vi "ModuleMain.vi"(8 "error in (no error)":errorcluster) -> (0 "error out":errorcluster)   [LabVIEW 2017, in "LeapMotion.lvlib"]
doc: "Module Main VI"
uses:
  LeapMotion.lvlib
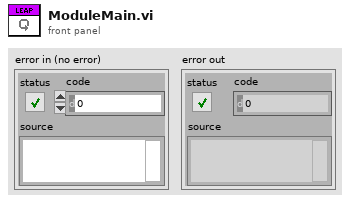
[diagram p1: front panel]
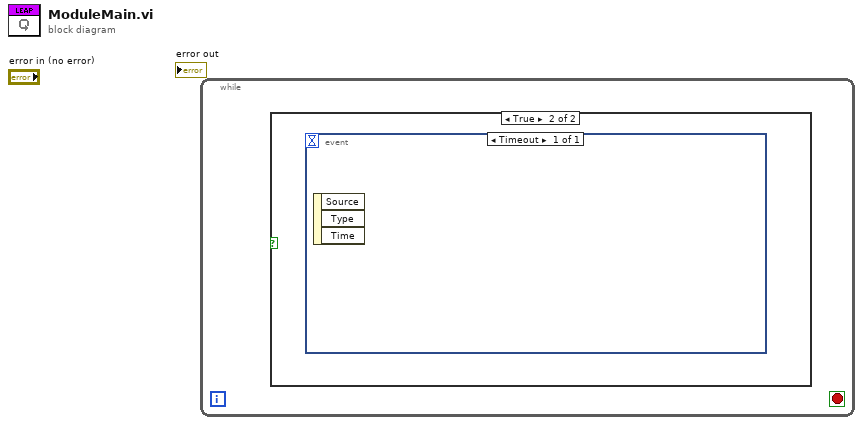
[diagram p0: block diagram]
diagram:
  n1 = while {
    stop <- _ stop-if-true
    n2 = case shown="True" {
      selector: _ -> [_ _]
      frame False {
      }
      frame True {
        n3 = event shown="[0] Timeout" {
          selector: _ -> [_]
          dyn-events: _ -> [_]
          timeout: _ -> [_]
          event Timeout {
            n4 = event-data() -> ()  [unwired: 1 in, 3 out]
          }
        }
      }
    }
  }
